vi "valueToImage.vi"(1 "variant":variant) -> (0 "Image":T1)   [LabVIEW 2015]
uses:
  <vilib>/vision/Image Controls.llb/IMAQ Image.ctl
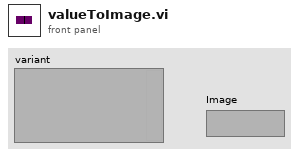
[diagram p1: front panel]
types:
  T1 = typedef "IMAQ Image.ctl" = refnum<image>
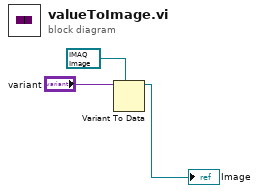
[diagram p0: block diagram]
diagram:
  n1 = Variant To Data(type=T1 refnum ("Image 2"), Variant="variant") -> (data=→"Image":T1)  [unwired: 1 in, 1 out]
